vi "init.vi"(0 "ConfigureILCMotorDriveStrategy in":refnum<class "ConfigureILCMotorDriveStrategy.lvclass">, 1 "LIMSW1 DAQ Channel To Write":refnum<k21>, 2 "LIMSW2 DAQ Channel To Write":refnum<k21>, 3 "Limit Switch Configuration":T1, 4 "MUX Settings":T3, 5 "error in (no error)":errorcluster) -> (14 "ConfigureILCMotorDriveStrategy out":refnum<class "ConfigureILCMotorDriveStrategy.lvclass">, 19 "error out":errorcluster)   [LabVIEW 2015, in "ConfigureILCMotorDriveStrategy.lvclass"]
uses:
  ConfigureILCMotorDriveStrategy.lvclass
  Typedefs/MUX Settings.ctl
  Typedefs/Digital Signal Level.ctl
  Typedefs/Limit Switch Configuration.ctl
  ConfigureILCMotorDriveStrategy.lvclass/ConfigureILCMotorDriveStrategy.ctl
  Typedefs/ILCBTTypedefs.lvlib
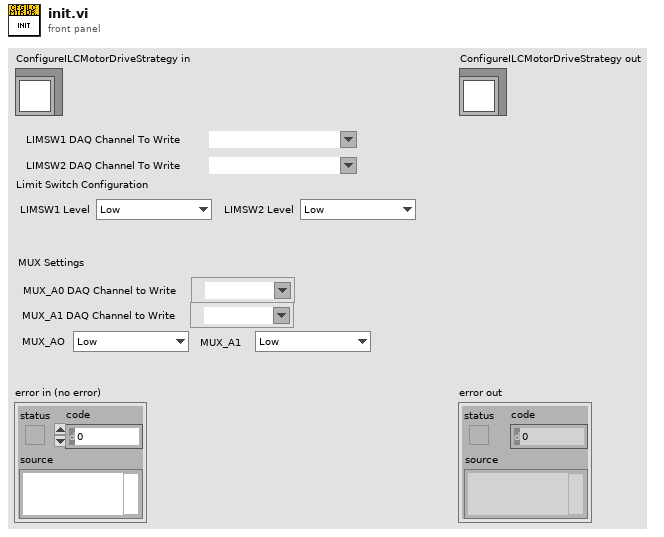
[diagram p1: front panel]
types:
  T1 = typedef "ILCBTTypedefs.lvlib/Limit Switch Configuration.ctl" = cluster{"LIMSW1 Level":T2, "LIMSW2 Level":T2}
  T2 = typedef "ILCBTTypedefs.lvlib/Digital Signal Level.ctl" = enum16{"Low", "High"}
  T3 = typedef "ILCBTTypedefs.lvlib/MUX Settings.ctl" = cluster{"MUX_AO":T2, "MUX_A1":T2, "MUX_A0 DAQ Channel to Write":refnum<k21>, "MUX_A1 DAQ Channel to Write":refnum<k21>}
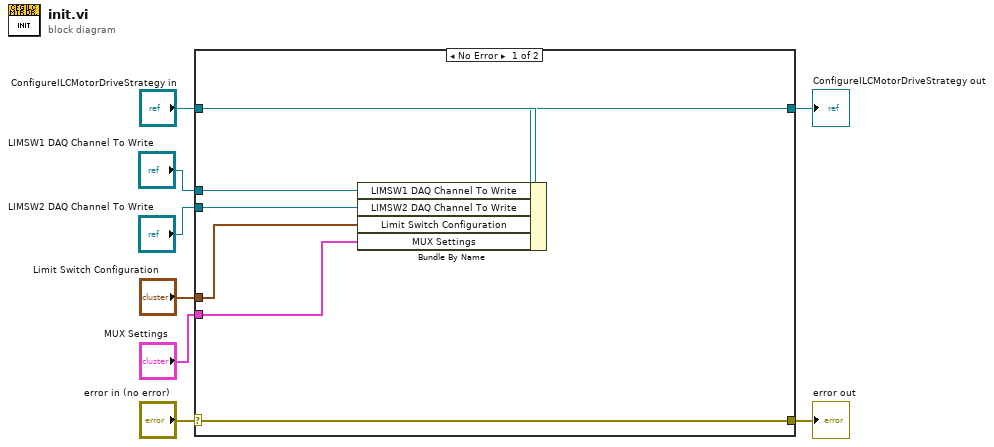
[diagram p0: block diagram]
diagram:
  n1 = case shown="No Error" "error in (no error)" {
    selector: "error in (no error)" -> [w15 w17]
    tunnel: [w15 w17] -> w7
    tunnel: [w13 w16] -> w5
    tunnel: "ConfigureILCMotorDriveStrategy in" -> [w14 w16]
    tunnel: "MUX Settings" -> [w12 _]
    tunnel: "Limit Switch Configuration" -> [w11 _]
    tunnel: "LIMSW1 DAQ Channel To Write" -> [w10 _]
    tunnel: "LIMSW2 DAQ Channel To Write" -> [w9 _]
    frame No Error {
      n2 = Bundle By Name(cluster=w14, "LIMSW1 DAQ Channel To Write"=w10, "LIMSW2 DAQ Channel To Write"=w9, "Limit Switch Configuration"=w11, "MUX Settings"=w12) -> (w13:refnum<class "ConfigureILCMotorDriveStrategy.lvclass">)
    }
    frame Error {
    }
  }
  "error out" <- w7
  "ConfigureILCMotorDriveStrategy out" <- w5
